vi "CST_Queue.vi"() -> (0 "Queue Cluster Element":T1)   [LabVIEW 2010]
uses:
  TYP_Queue Cluster Element.ctl
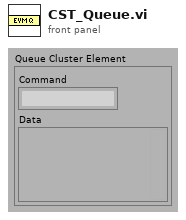
[diagram p1: front panel]
types:
  T1 = typedef "TYP_Queue Cluster Element.ctl" = cluster{"Command":string, "Data":variant}
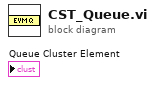
[diagram p0: block diagram]
diagram:
